vi "create bitmaps constats for zoom.vi"() -> ()   [LabVIEW 2014]
uses:
  <vilib>/picture/picture.llb/imagedata.ctl
panel:
  out "error out":errorcluster
  out "new picture":picture
  out "image data":T1
  out "new picture 2":picture
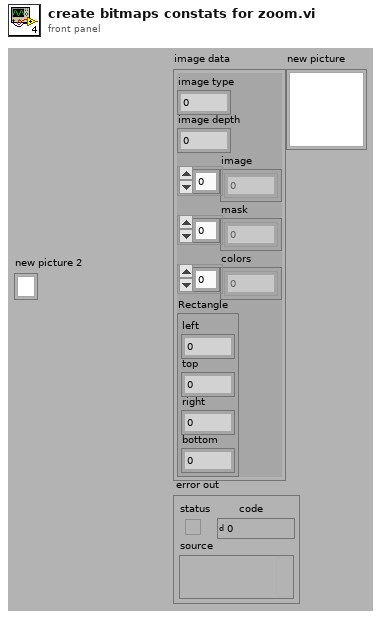
[diagram p1: front panel]
types:
  T1 = typedef "imagedata.ctl" = cluster{"image type":i32, "image depth":i32, "image":u8[], "mask":u8[], "colors":u32[], "Rectangle":cluster{"left":i16, "top":i16, "right":i16, "bottom":i16}}
  T2 = typedef "LVBoundsTypeDef.ctl" = cluster{"Width":u32, "Height":u32}
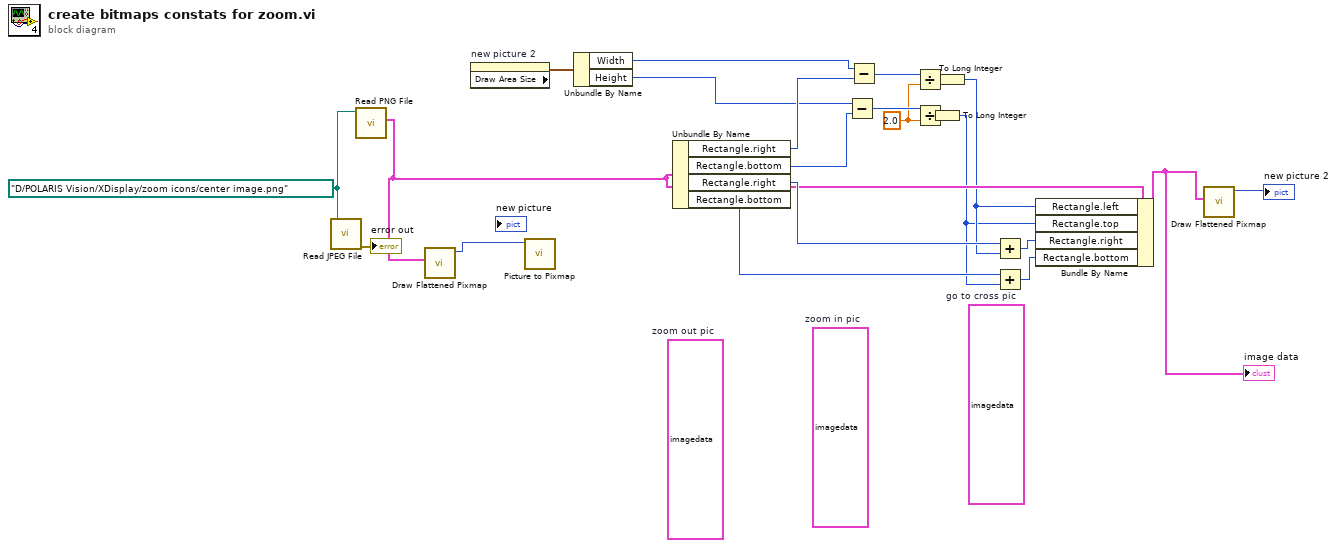
[diagram p0: block diagram]
diagram:
  (unwired) T1 {"image type"=0, "image depth"=32, "image"=[255, 246, 255, 255, 255, 246, 255, 255, 255, 251, 255, 255, 255, 249, 254, 248, 255, 255, 255, 251, 255, 255, 247, 243, 255, 146, 70, 72, 255, 255, 233, 234, 255, 255, 248, 245, 255, 254, 255, 253, 255, 255, 253, 255, 255, 255, 252, 255, 255, 255, 253, 255, 255, 252, 255, 255, 255, 250, 254, 255, 255, 249, 254, 250, 255, 251, 255, 251, 255, 244, 255, 249, 255, 255, 253, 241, 255, 124, 74, 63, 255, 255, 241, 230, 255, 255, 253, 243, 255, 251, 255, 251, 255, 255, 255, 255, 255, 255, 252, 255, 255, 255, 253, 254, 255, 255, 250, 255, 255, 255, 252, 254, 255, 255, 255, 253, 255, 242, 255, 247, 255, 227, 255, 246, 255, 104, 144, 110, 255, 129, 130, 96, 255, 129, 123, 91, 255, 248, 255, 237, 255, 233, 254, 237, 255, 249, 255, 251, 255, 255, 255, 253, 255, 254, 250, 247, 255, 255, 239, 247, 255, 255, 246, 248, 255, 255, 254, 244, 255, 249, 255, 241, 255, 105, 129, 103, 255, 243, 255, 227, 255, 107, 91, 57, 255, 255, 255, 220, 255, 112, 129, 97, 255, 244, 255, 241, 255, 255, 251, 242, 255, 255, 248, 246, 255, 255, 246, 246, 255, 255, 228, 237, 255, 255, 236, 235, 255, 255, 254, 228, 255, 132, 125, 96, 255, 255, 244, 228, 255, 255, 233, 227, 255, 166, 63, 56, 255, 255, 234, 216, 255, 255, 255, 225, 255, 124, 131, 100, 255, 255, 240, 236, 255, 255, 229, 238, 255, 255, 228, 238, 255, 146, 65, 74, 255, 132, 77, 74, 255, 94, 91, 60, 255, 123, 123, 89, 255, 131, 82, 68, 255, 152, 61, 60, 255, 174, 48, 51, 255, 163, 66, 57, 255, 95, 95, 59, 255, 115, 131, 95, 255, 130, 79, 75, 255, 147, 64, 74, 255, 153, 67, 80, 255, 255, 244, 249, 255, 255, 252, 248, 255, 242, 255, 239, 255, 111, 140, 109, 255, 252, 255, 239, 255, 255, 247, 236, 255, 155, 64, 63, 255, 255, 234, 225, 255, 243, 255, 228, 255, 97, 141, 105, 255, 255, 253, 241, 255, 255, 245, 248, 255, 255, 245, 251, 255, 255, 255, 255, 255, 245, 254, 249, 255, 239, 255, 245, 255, 234, 255, 243, 255, 100, 134, 110, 255, 254, 255, 239, 255, 127, 77, 66, 255, 255, 244, 228, 255, 109, 134, 104, 255, 227, 255, 243, 255, 248, 255, 250, 255, 255, 253, 252, 255, 255, 253, 255, 255, 251, 255, 255, 255, 248, 254, 250, 255, 254, 255, 253, 255, 249, 255, 250, 255, 235, 255, 243, 255, 111, 135, 109, 255, 128, 127, 96, 255, 127, 122, 92, 255, 247, 255, 241, 255, 244, 255, 250, 255, 251, 255, 253, 255, 255, 255, 253, 255, 255, 253, 251, 255, 246, 255, 250, 255, 254, 255, 253, 255, 255, 253, 255, 255, 255, 255, 253, 255, 245, 255, 250, 255, 245, 255, 239, 255, 95, 92, 61, 255, 255, 255, 228, 255, 255, 255, 246, 255, 251, 255, 255, 255, 252, 255, 255, 255, 254, 255, 255, 255, 255, 254, 250, 255, 254, 255, 251, 255, 252, 252, 250, 255, 255, 252, 253, 255, 255, 254, 255, 255, 253, 254, 249, 255, 255, 250, 243, 255, 127, 74, 66, 255, 255, 240, 236, 255, 255, 250, 250, 255, 252, 255, 255, 255, 251, 255, 255, 255, 251, 255, 255, 255, 254, 255, 251], "mask"=[255, 248, 255, 248, 255, 248, 255, 248, 255, 248, 255, 248, 255, 248, 255, 248, 255, 248, 255, 248, 255, 248], "colors"=[], "Rectangle"={"left"=0, "top"=0, "right"=13, "bottom"=11}}  # go to cross pic
  w6 = path "D:/POLARIS Vision/XDisplay/zoom icons/center image.png" ("path to JPEG file")
  (unwired) T1 {"image type"=0, "image depth"=24, "image"=[255, 255, 255, 255, 255, 255, 247, 255, 255, 231, 239, 247, 206, 214, 222, 189, 198, 214, 181, 189, 206, 165, 181, 198, 165, 181, 198, 206, 214, 222, 255, 255, 255, 247, 255, 255, 255, 255, 255, 255, 255, 255, 255, 255, 247, 255, 255, 247, 255, 255, 255, 247, 247, 255, 222, 222, 231, 206, 206, 222, 198, 214, 222, 206, 214, 231, 206, 222, 239, 198, 214, 231, 173, 181, 198, 132, 140, 156, 173, 181, 198, 255, 255, 255, 255, 255, 255, 255, 255, 255, 255, 255, 255, 255, 255, 247, 255, 255, 255, 231, 231, 247, 198, 206, 214, 206, 214, 231, 231, 239, 255, 231, 239, 255, 231, 247, 255, 222, 239, 255, 206, 222, 239, 165, 181, 198, 132, 140, 148, 198, 206, 214, 255, 255, 255, 255, 255, 255, 255, 247, 247, 255, 255, 255, 231, 239, 247, 198, 198, 214, 206, 214, 231, 231, 239, 255, 231, 247, 255, 214, 231, 255, 222, 239, 255, 231, 247, 255, 231, 247, 255, 214, 231, 255, 148, 156, 181, 148, 156, 173, 239, 247, 255, 255, 255, 255, 255, 255, 255, 255, 255, 255, 222, 222, 231, 173, 181, 189, 222, 231, 247, 231, 239, 255, 206, 222, 255, 206, 214, 255, 198, 206, 255, 189, 206, 255, 198, 214, 255, 214, 222, 255, 173, 181, 222, 132, 140, 173, 231, 239, 255, 255, 255, 255, 255, 255, 255, 255, 255, 255, 181, 189, 189, 165, 173, 181, 239, 247, 255, 198, 214, 239, 115, 123, 165, 99, 107, 156, 90, 99, 156, 74, 90, 148, 74, 90, 148, 198, 206, 255, 214, 222, 255, 132, 140, 173, 198, 206, 222, 255, 255, 255, 255, 255, 255, 255, 255, 247, 181, 198, 198, 148, 165, 165, 239, 247, 255, 231, 247, 255, 189, 206, 231, 198, 214, 239, 198, 214, 247, 189, 206, 239, 189, 198, 239, 214, 222, 255, 198, 206, 231, 148, 156, 173, 214, 222, 231, 247, 255, 255, 255, 255, 255, 255, 255, 255, 231, 239, 231, 148, 156, 156, 206, 214, 214, 247, 255, 255, 247, 255, 255, 247, 255, 255, 239, 255, 255, 239, 247, 255, 231, 247, 255, 222, 239, 255, 189, 198, 214, 156, 173, 173, 239, 247, 247, 255, 255, 255, 255, 255, 255, 255, 255, 247, 247, 255, 255, 189, 198, 198, 148, 156, 156, 247, 255, 255, 247, 255, 255, 247, 255, 255, 247, 255, 255, 239, 247, 255, 239, 247, 255, 206, 222, 231, 173, 181, 189, 198, 206, 206, 255, 255, 255, 255, 255, 255, 255, 255, 255, 255, 255, 247, 255, 255, 255, 247, 255, 255, 165, 165, 173, 148, 156, 156, 214, 222, 231, 255, 255, 255, 239, 247, 255, 231, 239, 247, 206, 214, 222, 173, 181, 189, 148, 156, 156, 206, 214, 214, 247, 247, 247, 247, 247, 247, 255, 255, 255, 255, 255, 255, 255, 255, 255, 255, 255, 255, 247, 247, 255, 189, 189, 198, 148, 148, 165, 156, 165, 173, 189, 189, 206, 181, 181, 198, 181, 181, 198, 189, 198, 206, 173, 173, 181, 123, 123, 132, 123, 123, 123, 247, 247, 255, 255, 255, 255, 255, 255, 255, 255, 255, 255, 255, 255, 255, 255, 255, 255, 255, 255, 255, 231, 231, 239, 222, 222, 231, 206, 214, 222, 214, 222, 231, 239, 239, 247, 255, 255, 255, 222, 222, 239, 140, 140, 148, 82, 82, 82, 115, 107, 115, 247, 239, 247, 255, 255, 255, 255, 255, 255, 255, 255, 255, 255, 255, 255, 255, 255, 255, 255, 255, 255, 255, 255, 255, 255, 255, 255, 255, 255, 255, 255, 255, 255, 255, 255, 255, 255, 255, 255, 206, 206, 206, 148, 148, 148, 82, 82, 82, 132, 123, 132, 231, 231, 239, 255, 255, 255, 255, 255, 255, 255, 255, 255, 247, 247, 247, 255, 255, 255, 255, 255, 255, 255, 255, 255, 255, 255, 255, 255, 255, 247, 255, 255, 255, 255, 255, 247, 255, 255, 255, 198, 198, 198, 148, 148, 148, 82, 74, 82, 156, 156, 156, 255, 255, 255, 255, 255, 255, 255, 255, 255, 255, 255, 255, 255, 255, 255, 255, 255, 255, 255, 255, 255, 255, 255, 255, 255, 255, 255, 255, 255, 255, 255, 255, 255, 255, 255, 255, 255, 255, 255, 206, 206, 206, 148, 148, 148, 214, 222, 214, 255, 255, 255, 255, 255, 247, 255, 255, 255, 255, 255, 255, 255, 255, 255, 255, 255, 255, 255, 255, 255, 255, 255, 255, 255, 255, 255, 255, 255, 255, 255, 255, 255, 255, 255, 255, 255, 255, 255, 255, 255, 255, 255, 255, 247, 255, 255, 255], "mask"=[], "colors"=[], "Rectangle"={"left"=0, "top"=0, "right"=16, "bottom"=16}}  # zoom out pic
  (unwired) T1 {"image type"=0, "image depth"=24, "image"=[255, 255, 247, 255, 255, 247, 247, 255, 255, 231, 239, 239, 206, 214, 222, 181, 198, 214, 181, 189, 206, 165, 189, 198, 165, 181, 189, 198, 214, 214, 247, 255, 255, 247, 255, 247, 255, 255, 255, 255, 255, 255, 255, 247, 255, 255, 255, 255, 255, 255, 255, 247, 255, 247, 214, 222, 231, 189, 198, 214, 198, 206, 222, 214, 231, 255, 198, 214, 239, 189, 214, 231, 173, 189, 206, 123, 140, 148, 173, 181, 189, 255, 255, 255, 255, 255, 255, 255, 255, 255, 255, 255, 255, 255, 255, 255, 247, 255, 255, 231, 239, 239, 189, 198, 214, 214, 222, 247, 231, 239, 255, 222, 239, 255, 206, 222, 255, 222, 239, 255, 206, 222, 255, 165, 181, 206, 123, 140, 156, 198, 206, 214, 255, 255, 255, 255, 255, 255, 255, 247, 255, 255, 255, 255, 247, 247, 255, 189, 198, 206, 206, 214, 239, 231, 239, 255, 231, 239, 255, 189, 206, 255, 115, 132, 181, 198, 214, 255, 231, 247, 255, 214, 231, 255, 140, 156, 181, 148, 156, 173, 239, 247, 255, 255, 255, 255, 255, 255, 255, 255, 255, 255, 222, 231, 239, 173, 181, 198, 222, 231, 255, 222, 231, 255, 206, 222, 255, 165, 181, 239, 90, 107, 165, 181, 198, 255, 198, 214, 255, 206, 222, 255, 165, 181, 214, 132, 140, 165, 231, 239, 247, 247, 255, 255, 255, 255, 255, 255, 255, 255, 198, 198, 206, 173, 173, 189, 239, 247, 255, 198, 206, 247, 115, 123, 173, 99, 115, 173, 82, 99, 156, 66, 90, 148, 74, 90, 148, 189, 214, 255, 206, 222, 255, 132, 140, 165, 198, 206, 222, 255, 255, 255, 255, 255, 255, 255, 255, 255, 206, 206, 214, 156, 156, 173, 231, 239, 255, 231, 239, 255, 198, 214, 255, 156, 173, 214, 66, 82, 132, 165, 189, 231, 181, 206, 247, 206, 231, 255, 189, 206, 231, 148, 156, 173, 214, 222, 222, 255, 255, 255, 255, 255, 255, 255, 255, 255, 239, 239, 239, 148, 148, 156, 214, 214, 231, 247, 255, 255, 247, 255, 255, 198, 214, 239, 82, 99, 132, 198, 222, 255, 231, 247, 255, 214, 239, 255, 181, 198, 214, 156, 173, 181, 239, 247, 255, 255, 255, 255, 255, 255, 255, 255, 255, 247, 255, 255, 255, 189, 189, 198, 148, 156, 165, 239, 247, 255, 247, 255, 255, 231, 247, 255, 189, 206, 231, 231, 247, 255, 231, 247, 255, 206, 222, 231, 173, 181, 189, 198, 206, 214, 247, 255, 255, 255, 255, 255, 255, 255, 255, 255, 255, 255, 255, 255, 255, 239, 239, 239, 165, 173, 173, 148, 148, 156, 206, 222, 222, 247, 255, 255, 231, 247, 255, 231, 247, 255, 206, 214, 222, 173, 181, 189, 140, 156, 156, 206, 214, 214, 247, 247, 247, 247, 247, 247, 255, 255, 255, 255, 255, 255, 255, 255, 255, 255, 255, 255, 247, 247, 255, 181, 189, 189, 148, 156, 156, 156, 165, 165, 181, 189, 198, 173, 189, 189, 181, 189, 189, 189, 198, 206, 165, 173, 181, 123, 123, 132, 123, 123, 123, 247, 247, 255, 255, 255, 255, 255, 255, 255, 255, 255, 255, 255, 255, 255, 255, 255, 255, 255, 255, 255, 231, 231, 231, 214, 222, 214, 214, 214, 214, 214, 214, 222, 239, 239, 247, 255, 255, 255, 222, 222, 231, 148, 140, 148, 82, 82, 90, 115, 107, 115, 247, 239, 247, 255, 255, 255, 255, 255, 255, 255, 255, 255, 255, 255, 255, 255, 255, 255, 255, 255, 255, 255, 255, 255, 255, 255, 255, 255, 255, 255, 255, 255, 255, 255, 255, 255, 255, 255, 255, 206, 206, 214, 148, 148, 156, 82, 82, 90, 132, 123, 132, 231, 231, 239, 255, 255, 255, 255, 255, 255, 255, 255, 255, 255, 255, 255, 247, 247, 247, 255, 255, 255, 255, 255, 255, 255, 255, 255, 255, 255, 255, 255, 255, 255, 255, 255, 255, 255, 255, 255, 198, 198, 206, 148, 148, 148, 74, 74, 74, 156, 156, 156, 255, 255, 255, 255, 255, 255, 255, 255, 255, 255, 255, 255, 255, 255, 255, 255, 255, 255, 255, 255, 255, 255, 255, 255, 255, 255, 255, 255, 255, 255, 255, 255, 255, 255, 255, 255, 255, 255, 255, 206, 206, 206, 148, 148, 140, 214, 222, 206, 255, 255, 255, 255, 255, 255, 255, 255, 255, 255, 255, 255, 255, 255, 255, 255, 255, 255, 255, 255, 255, 255, 255, 255, 255, 255, 255, 255, 255, 255, 255, 255, 255, 255, 255, 255, 255, 255, 255, 255, 255, 255, 247, 255, 239, 255, 255, 247], "mask"=[], "colors"=[], "Rectangle"={"left"=0, "top"=0, "right"=16, "bottom"=16}}  # zoom in pic
  w15 = 2.0 ("y")
  n1 = call <vilib>:"Read JPEG File.vi"("path to JPEG file"=w6) -> ("error out"=→"error out":errorcluster)  [unwired: 8 in, 2 out]
  n2 = call <vilib>:"Read PNG File.vi"("path to PNG file"=w6) -> ("image data"=w5:T1)  [unwired: 8 in, 2 out]
  n3 = call <vilib>:"Draw Flattened Pixmap.vi"("image data"=w5) -> ("new picture"=w7:picture)  [unwired: 8 in]
  n4 = property on="new picture 2" class="Pict"() -> ("Draw Area Size"=w22:T2)  [unwired: 2 in, 2 out]
  n5 = call <vilib>:"Picture to Pixmap.vi"("picture"=w7) -> ()  [unwired: 9 in, 2 out]
  n6 = Unbundle By Name(w22) -> ("Width"=w21:u32, "Height"=w19:u32)
  n7 = Unbundle By Name(w5) -> ("Rectangle.right"=w20:i16, "Rectangle.bottom"=w17:i16, "Rectangle.right"=w14:i16, "Rectangle.bottom"=w11:i16)
  n8 = Subtract(x=w19, y=w17) -> (x-y=w16:u32)
  n9 = Subtract(x=w21, y=w20) -> (x-y=w18:u32)
  n10 = Divide(x=w18, y=w15) -> (x/y=w13:dbl)
  n11 = Divide(x=w16, y=w15) -> (x/y=w10:dbl)
  n12 = To Long Integer(number=w10) -> (32bit integer=w1:i32)
  n13 = To Long Integer(number=w13) -> (32bit integer=w2:i32)
  n14 = Add(x=w14, y=w2) -> (x+y=w12:i32)
  n15 = Add(x=w11, y=w1) -> (x+y=w9:i32)
  n16 = Bundle By Name(cluster=w5, "Rectangle.left"=w2, "Rectangle.top"=w1, "Rectangle.right"=w12, "Rectangle.bottom"=w9) -> (w3:T1)
  "image data" <- w3
  n17 = call <vilib>:"Draw Flattened Pixmap.vi"("image data"=w3) -> ("new picture"=→"new picture 2":picture)  [unwired: 8 in]
